vi "Retry Timeout.vi"(8 "error in (no error)":errorcluster, 10 "time (s) [10 s]":dbl=10.0, 11 "reset":bool) -> (0 "error out":errorcluster, 3 "Timeout?":bool)   [LabVIEW 2019, in "Instrument.Lockin.lvclass"]
uses:
  Instrument.Lockin.lvclass
  <vilib>/Utility/error.llb/Error Cluster From Error Code.vi
  <vilib>/ErrorRing/Error Ring.xnode
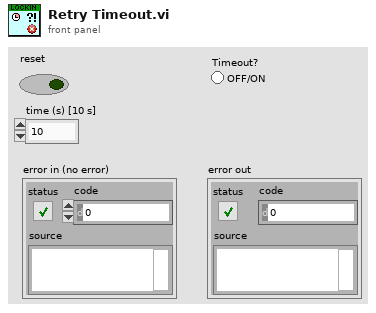
[diagram p1: front panel]
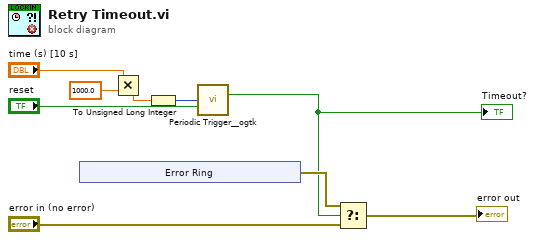
[diagram p0: block diagram]
diagram:
  n1 = xnode "Error Ring"() -> ("error out"=w7:errorcluster)
  n2 = Multiply(x="time (s) [10 s]", y=1000.0) -> (x*y=w3:dbl)
  n3 = To Unsigned Long Integer(number=w3) -> (unsigned 32bit integer=w1:u32)
  n4 = call <userlib>:"Periodic Trigger__ogtk.vi"("time (ms)"=w1, "reset"="reset") -> ("Triggered"=w6:bool)  [unwired: 11 in, 2 out]
  "Timeout?" <- w6
  n5 = Select(t=w7, s=w6, f="error in (no error)") -> (s? t:f=→"error out":errorcluster)
